vi "To TCP Config.vi"(5 "Wifi Configuration":T1) -> (2 "TCP Configuration":T3)   [LabVIEW 2019, in "LINXx.lvlib"]
doc: "Extracts TCP configuration from WiFi configuration"
uses:
  LINXx.lvlib
  <vilib>/MakerHub/LINX/Private/Device/Type Defs/TCP Config.ctl
  <vilib>/MakerHub/LINX/Private/Device/Type Defs/Wifi Config.ctl
  <vilib>/MakerHub/LINX/Private/Type Defs/WIFI Security Type.ctl
  <vilib>/MakerHub/LINX/Private/Device/Device.lvlib
  <vilib>/MakerHub/LINX/LMH-LINX.lvlib
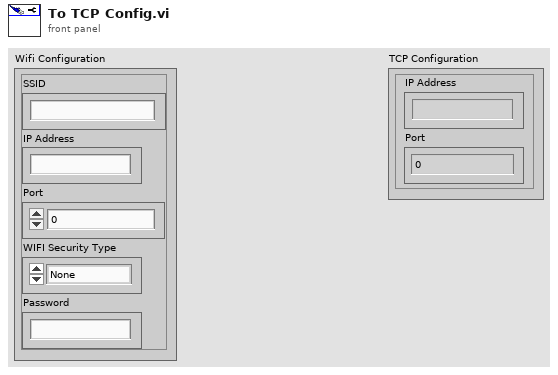
[diagram p1: front panel]
types:
  T1 = typedef "LMH-LINX.lvlib/Device.lvlib/Wifi Config.ctl" = cluster{"SSID":string, "IP Address":string, "Port":u16, "WIFI Security Type":T2, "Password":string}
  T2 = typedef "LMH-LINX.lvlib/WIFI Security Type.ctl" = enum8{"None", "WPA2 Password", "WPA2 Key", "WEP40", "WEP104"}
  T3 = typedef "LMH-LINX.lvlib/Device.lvlib/TCP Config.ctl" = cluster{"IP Address":string, "Port":u16}
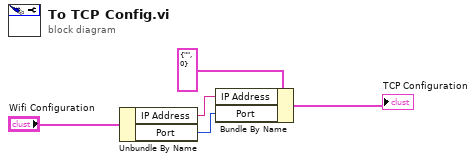
[diagram p0: block diagram]
diagram:
  n1 = Unbundle By Name("Wifi Configuration") -> ("IP Address"=w3:string, "Port"=w2:u16)
  n2 = Bundle By Name(cluster=T3 {"IP Address"="", "Port"=0} ("TCP Configuration"), "IP Address"=w3, "Port"=w2) -> (→"TCP Configuration":T3)
